vi "Check_State.vi"(0 "object in":refnum<class "Navigation.lvclass">, 5 "error in (no error)":errorcluster) -> (14 "object out":refnum<class "Navigation.lvclass">, 19 "error out":errorcluster)   [LabVIEW 2023, in "Navigation.lvclass"]
uses:
  Navigation.lvclass
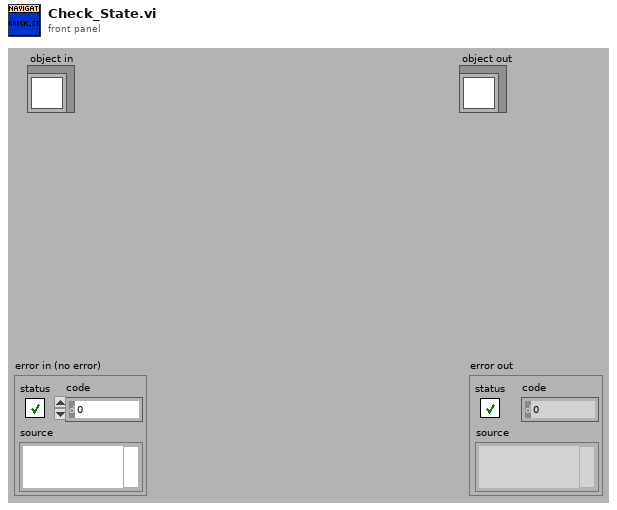
[diagram p1: front panel]
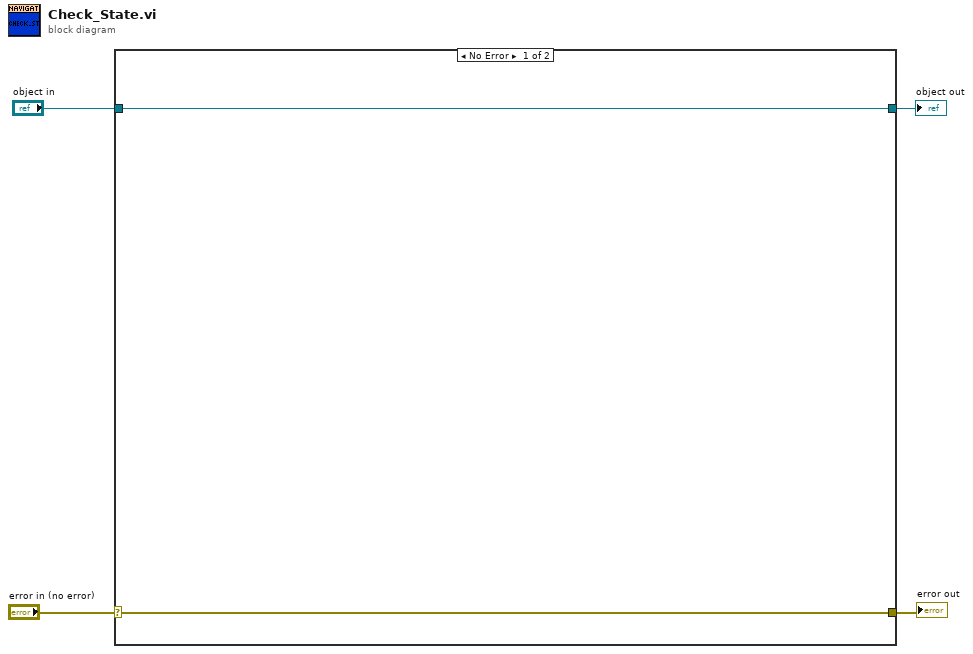
[diagram p0: block diagram]
diagram:
  n1 = case shown="No Error" "error in (no error)" {
    selector: "error in (no error)" -> [w5 w8]
    tunnel: [w5 w8] -> w3
    tunnel: [w6 w7] -> w1
    tunnel: "object in" -> [w6 w7]
    frame No Error {
    }
    frame Error {
    }
  }
  "error out" <- w3
  "object out" <- w1
